vi "SummaryWithGlyphManager.vi"(8 "error in":errorcluster, 9 "glyph manager":T1, 10 "depth":i32, 11 "node self ref":T3) -> (0 "error out":errorcluster, 1 "glyph manager out":T1, 2 "summary":T4[](array[typedef]))   [LabVIEW 2013, in "NISE_CEF_TreeControl.lvlib"]
doc: "Gets the summary of a node and all the subnodes. This description can be used to update the tree control"
uses:
  NISE_CEF_TreeControl.lvlib
  Node/Summary.ctl
  Node/NodeRef.ctl
  Node/NISE_CEF_Node.lvclass
  glyph manager/glyph manager.ctl
  <vilib>/picture/picture.llb/imagedata.ctl
  Node/NISE_CEF_Node.lvclass/NISE_CEF_Node.ctl
  Node/ReadParent.vi
  Node/ReadChildren.vi
  Node/ReadNodeClass.vi
  glyph manager/glyph manager.lvlib
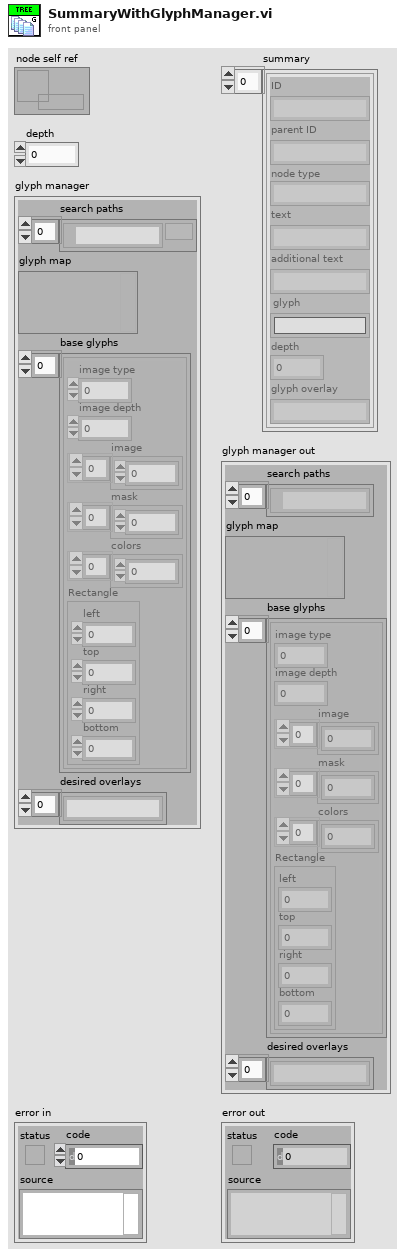
[diagram p1: front panel]
types:
  T1 = typedef "glyph manager.lvlib/glyph manager.ctl" = cluster{"search paths":path[], "glyph map":variant, "base glyphs":T2[], "desired overlays":string[]}
  T2 = typedef "imagedata.ctl" = cluster{"image type":i32, "image depth":i32, "image":u8[], "mask":u8[], "colors":u32[], "Rectangle":cluster{"left":i16, "top":i16, "right":i16, "bottom":i16}}
  T3 = typedef "NISE_CEF_Node.lvclass/NodeRef.ctl" = refnum<data-value>
  T4 = typedef "NISE_CEF_Node.lvclass/Summary.ctl" = cluster{"ID":string, "parent ID":string, "node type":string, "text":string, "additional text":string, "glyph":string, "depth":i32, "glyph overlay":string}
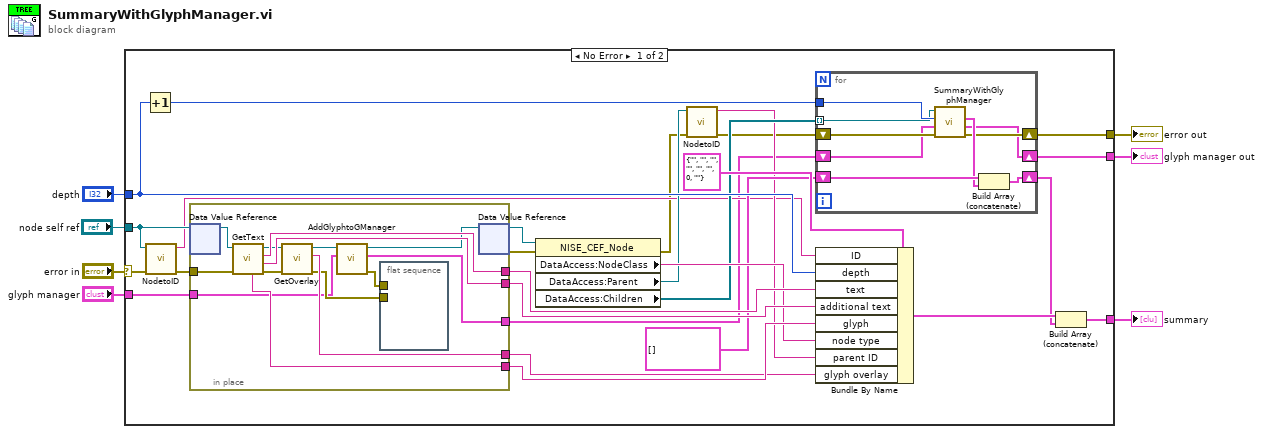
[diagram p0: block diagram]
diagram:
  n1 = case shown="No Error" "error in" {
    selector: "error in" -> [w18 w59]
    tunnel: [w12 w59] -> w6
    tunnel: "node self ref" -> [w20 _]
    tunnel: "depth" -> [w34 _]
    tunnel: [w33 _] -> w3
    tunnel: "glyph manager" -> [w10 w58]
    tunnel: [w8 w58] -> w1
    frame No Error {
      n2 = Increment(x=w34) -> (x+1=w27:i32)
      n3 = call "NodetoID.vi"("error in"=w18, "node ref"=w20) -> ("error out"=w17:errorcluster, "ID"=w19:string)  [unwired: 8 in]
      n4 = in-place {
        in-place-border: [w48] -> w31
        in-place-border: [w47] -> w30
        in-place-border: [w46] -> w29
        in-place-border: w17 -> [w45]
        in-place-border: [w41] -> w11
        in-place-border: w10 -> [w36]
        in-place-border: [w35] -> w9
        n5 = in-place-dvr #1(w20) -> (w44:refnum<class "NISE_CEF_Node.lvclass">)  [unwired: 1 out]
        n6 = call-dynamic "GetText.vi"("error in"=w45, "node in"=w44) -> ("error out"=w42:errorcluster, "additional text"=w48:string, "text"=w47:string, "node out"=w43:refnum<class "NISE_CEF_Node.lvclass">, "glyph"=w46:string)  [unwired: 5 in]
        n7 = call-dynamic "GetOverlay.vi"("error in"=w42, "NISE_CEF_Node in"=w43) -> ("error out"=w37:errorcluster, "overlay"=w41:string, "NISE_CEF_Node out"=w40:refnum<class "NISE_CEF_Node.lvclass">)  [unwired: 7 in]
        n8 = call-dynamic "AddGlyphtoGManager.vi"("glyph manager"=w36, "NISE_CEF_Node in"=w40) -> ("error out"=w38:errorcluster, "glyph manager out"=w35:T1, "NISE_CEF_Node out"=w39:refnum<class "NISE_CEF_Node.lvclass">)  [unwired: 7 in]
        n9 = flat-sequence {
          tunnel: w38 -> [_]
          tunnel: w37 -> [_]
          frame #0 {
          }
        }
        n10 = in-place-dvr #1(w39) -> (w16:T3, w15:errorcluster)
      }
      n11 = property class="NISE_CEF_Node"(reference=w16, error in=w15) -> (error out=w14:errorcluster, "DataAccess:NodeClass"=w28:string, "DataAccess:Parent"=w22:T3, "DataAccess:Children"=w23:T3[])  [unwired: 1 out]
      n12 = call "NodetoID.vi"("error in"=w14, "node ref"=w22) -> ("error out"=w13:errorcluster, "ID"=w21:string)  [unwired: 8 in]
      n13 = for {
        tunnel: w23 -> [w53] mode=indexing
        tunnel: w27 -> [w57]
        shift-right: [w55] -> w24
        shift-left: T4[] [] ("childrensummary") -> [w56]
        shift-right: [w51] -> w12
        shift-left: w13 -> [w52]
        shift-right: [w49] -> w8
        shift-left: w9 -> [w50]
        n14 = call "SummaryWithGlyphManager.vi"("error in"=w52, "glyph manager"=w50, "depth"=w57, "node self ref"=w53) -> ("error out"=w51:errorcluster, "glyph manager out"=w49:T1, "summary"=w54:T4[])  [unwired: 5 in]
        n15 = Build Array (concatenate)(w56, w54) -> (w55:T4[])
      }
      n16 = Bundle By Name(cluster=T4 {"ID"="", "parent ID"="", "node type"="", "text"="", "additional text"="", "glyph"="", "depth"=0, "glyph overlay"=""} ("nodeSummary"), "ID"=w19, "depth"=w34, "text"=w30, "additional text"=w31, "glyph"=w29, "node type"=w28, "parent ID"=w21, "glyph overlay"=w11) -> (w25:T4)
      n17 = Build Array (concatenate)(w25, w24) -> (w33:T4[])
    }
    frame Error {
    }
  }
  "error out" <- w6
  "summary" <- w3
  "glyph manager out" <- w1
